vi "Close.vi"(7 "Abort (F)":bool, 8 "error in (no error)":errorcluster, 11 "Event in":refnum<class "Event.lvclass">) -> (0 "error out":errorcluster)   [LabVIEW 2022 SP3, in "Enclave.lvlib" / "Event.lvclass"]
uses:
  Event.lvclass
  Event.lvclass/Event.ctl
  Enclave/Enclave.lvclass
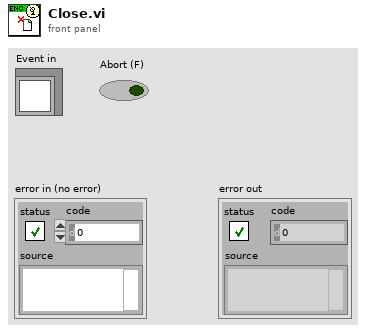
[diagram p1: front panel]
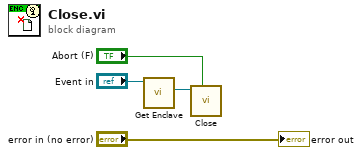
[diagram p0: block diagram]
diagram:
  n1 = call "Get Enclave.vi"("Event in"="Event in") -> ("Enclave"=w2:refnum<class "Enclave.lvclass">)  [unwired: 8 in, 2 out]
  n2 = call "Close.vi"("Abort (F)"="Abort (F)", "Enclave in"=w2) -> ()  [unwired: 9 in, 1 out]
  "error out" <- "error in (no error)"
